vi "Actor Core.vi"(8 "error in":errorcluster, 11 "Filled Text Fields Actor in":refnum<class "Filled Text Fields Actor.lvclass">) -> (0 "error out":errorcluster, 3 "Actor out":refnum<class "Actor.lvclass">)   [LabVIEW 2017, in "Filled Text Fields Actor.lvlib" / "Filled Text Fields Actor.lvclass"]
doc: "(<B>Filename</B>: Actor Framework.lvlib:Actor.lvclass:Actor Core.vi)\n\nReceives messages to the actor, reacts to them, and initiates any error handling that may shut the actor down.\n\nDescendant classes may override this VI to append parallel tasks for the actor to complete while it handles messages. Overrides use the Call Parent Method node."
uses:
  Filled Text Fields Actor.lvclass
  <vilib>/ActorFramework/Actor/Actor.lvclass
  Filled Text Fields Actor.lvclass/Filled Text Fields Actor.ctl
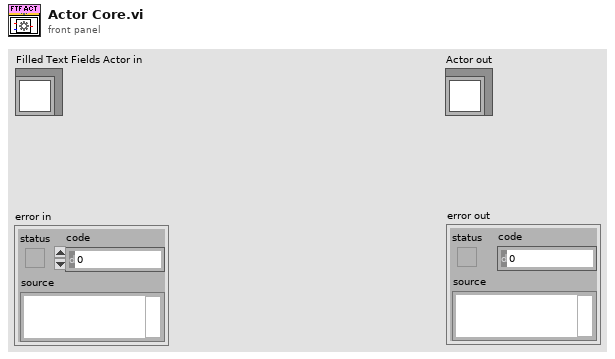
[diagram p1: front panel]
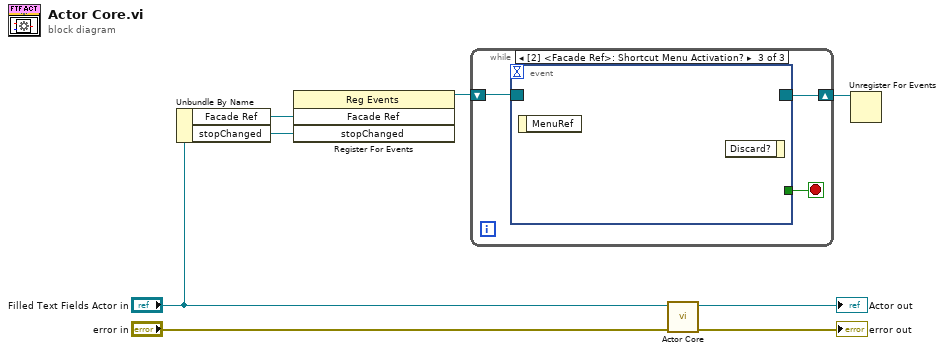
[diagram p0: block diagram]
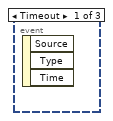
[diagram p2: hidden frame]
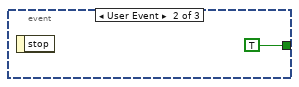
[diagram p3: hidden frame]
diagram:
  n1 = Unbundle By Name("Filled Text Fields Actor in") -> ("Facade Ref"=w3:refnum<vi>, "stopChanged"=w2:refnum<user-event>)
  n2 = register-events(w3, w2) -> (reference out=w4:refnum<event-registration>)  [unwired: 2 in, 1 out]
  n3 = while {
    shift-right: [w10] -> w1
    shift-left: w4 -> [w11]
    stop <- w9 stop-if-true
    n4 = event shown="[2] <Facade Ref>: Shortcut Menu Activation?" {
      selector: w11 -> [_ _ _]
      dyn-events: [_ _ _] -> w10
      timeout: _ -> [_ _ _]
      tunnel: [_ TRUE _] -> w9
      event Timeout {
        n5 = event-data() -> ()  [unwired: 1 in, 3 out]
      }
      event User Event {
        n6 = event-data() -> ()  [unwired: 1 in, 1 out]
      }
      event Shortcut Menu Activation? {
        n7 = event-data() -> ()  [unwired: 1 in, 1 out]
        n8 = event-data() -> ()  [unwired: 2 in, 1 out]
      }
    }
  }
  n9 = call-parent "Actor Core.vi"("error in"="error in", "Actor in"="Filled Text Fields Actor in") -> ("error out"=→"error out":errorcluster, "Actor out"=→"Actor out":refnum<class "Actor.lvclass">)  [unwired: 8 in]
  n10 = Unregister For Events(event registration refnum=w1) -> ()  [unwired: 1 in, 1 out]
